vi "Load_Cell_Calcs.vi"(0 "VFz - Load Cell 1":dbl, 1 "VFy - Load Cell 2":dbl, 2 "VFx - Load Cell 3":dbl, 3 "VFz - Load Cell 4":dbl, 4 "VFy - Load Cell 4":dbl, 5 "VFx - Load Cell 1":dbl, 7 "VFy - Load Cell 1":dbl, 9 "VFz - Load Cell 2":dbl, 11 "VFx - Load Cell 2":dbl, 12 "VFz - Load Cell 3":dbl, 13 "VFy - Load Cell 3":dbl, 14 "VFx - Load Cell 4":dbl) -> (6 "Fz":dbl, 8 "Fx":dbl, 10 "Fy":dbl)   [LabVIEW 2025]
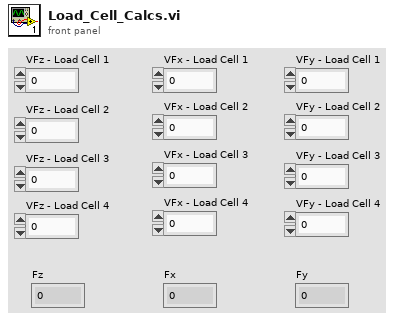
[diagram p1: front panel]
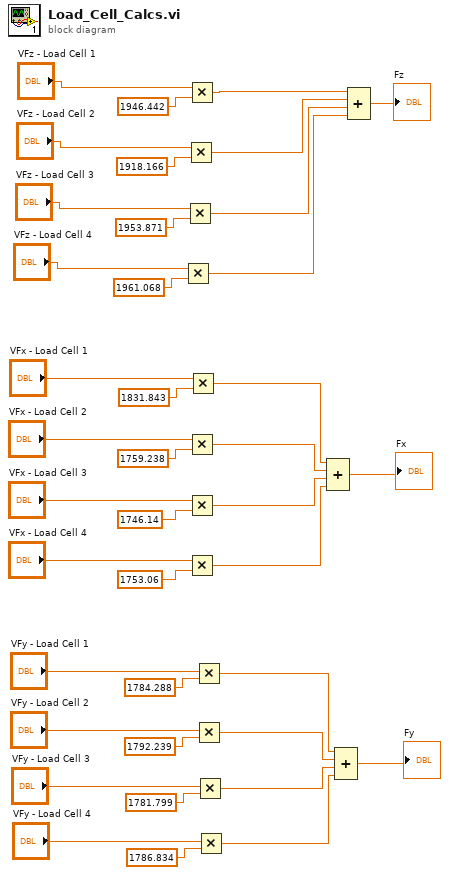
[diagram p0: block diagram]
diagram:
  n1 = Multiply(x="VFz - Load Cell 4", y=1961.068) -> (x*y=w12:dbl)
  n2 = Multiply(x="VFz - Load Cell 3", y=1953.871) -> (x*y=w13:dbl)
  n3 = Multiply(x="VFz - Load Cell 2", y=1918.166) -> (x*y=w14:dbl)
  n4 = Multiply(x="VFz - Load Cell 1", y=1946.442) -> (x*y=w15:dbl)
  n5 = Multiply(x="VFx - Load Cell 2", y=1759.238) -> (x*y=w8:dbl)
  n6 = Multiply(x="VFx - Load Cell 3", y=1746.14) -> (x*y=w7:dbl)
  n7 = Multiply(x="VFx - Load Cell 4", y=1753.06) -> (x*y=w6:dbl)
  n8 = Multiply(x="VFx - Load Cell 1", y=1831.843) -> (x*y=w9:dbl)
  n9 = Multiply(x="VFy - Load Cell 1", y=1784.288) -> (x*y=w4:dbl)
  n10 = Multiply(x="VFy - Load Cell 2", y=1792.239) -> (x*y=w3:dbl)
  n11 = Multiply(x="VFy - Load Cell 3", y=1781.799) -> (x*y=w2:dbl)
  n12 = Multiply(x="VFy - Load Cell 4", y=1786.834) -> (x*y=w1:dbl)
  n13 = Compound Arithmetic op=ADD(w9, w8, w7, w6) -> (→"Fx":dbl)
  n14 = Compound Arithmetic op=ADD(w4, w3, w2, w1) -> (→"Fy":dbl)
  n15 = Compound Arithmetic op=ADD(w15, w14, w13, w12) -> (→"Fz":dbl)
